vi "CRC_TESTED.vi"() -> ()   [LabVIEW 2019]
panel:
  out "Numeric 7":u16 format="%b"
  out "Numeric":u16 format="%b"
  out "CRC =   5":u16 format="%x"
  out "CRC =   4":u16 format="%b"
  out "CRC =   3":u16 format="%b"
  out "CRC =   2":u16 format="%x"
  in  "DATA PACKET":string
  out "CRC =":u16 format="%x"
  # "1100 0110 1100 1100"
  # "Polynom X16+X12+X5+1"
  # "Felica and 14443 Type A - GOOD"
  # "15693 and 14443 Type B"
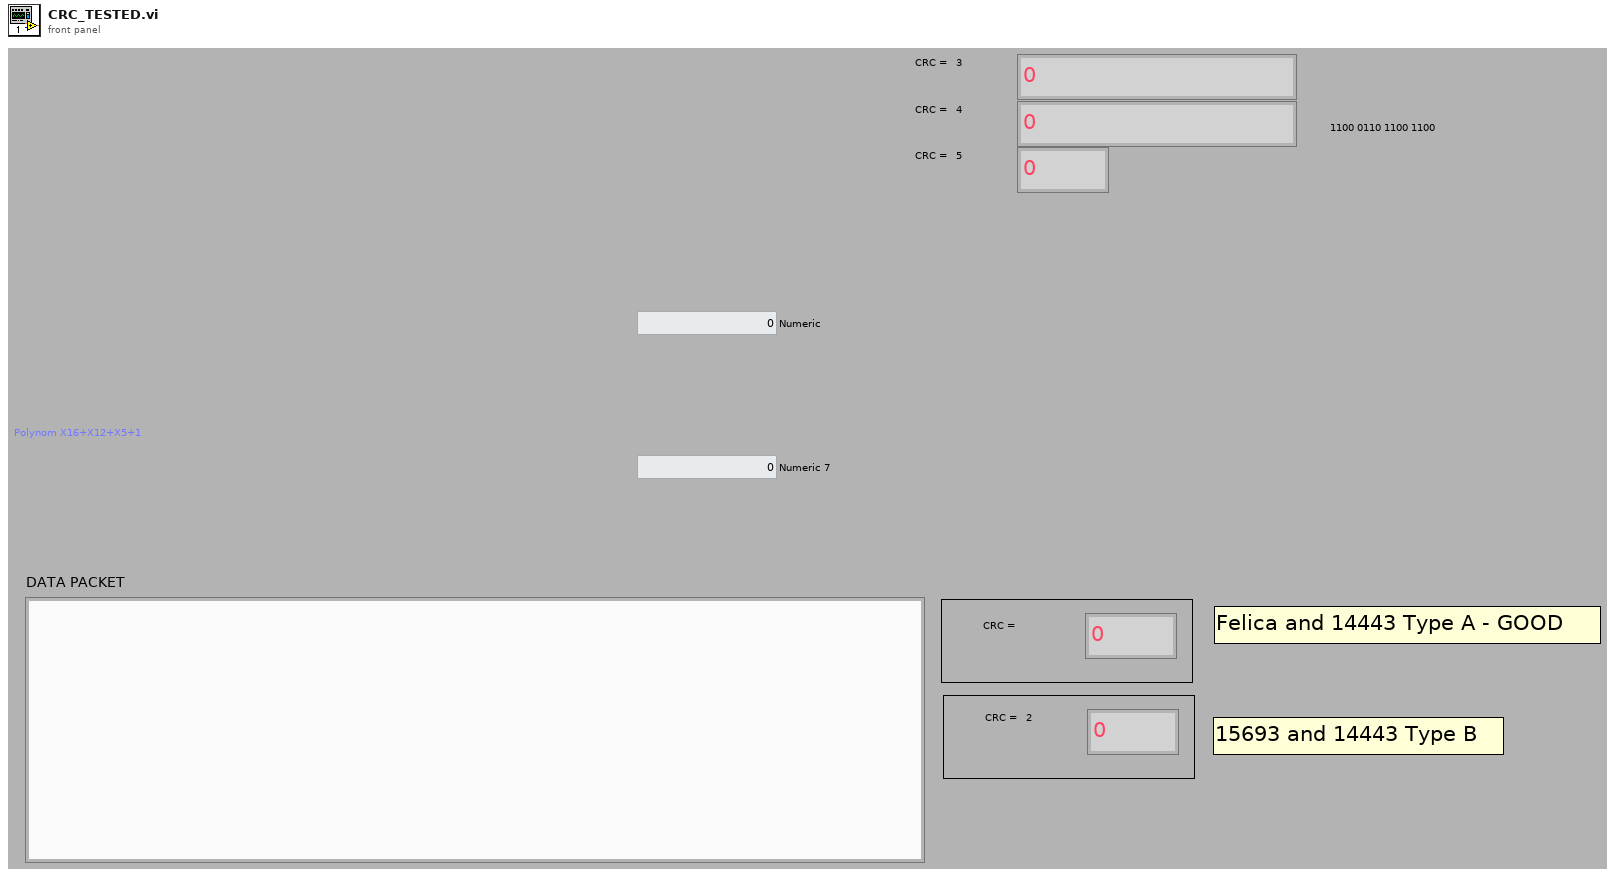
[diagram p1: front panel]
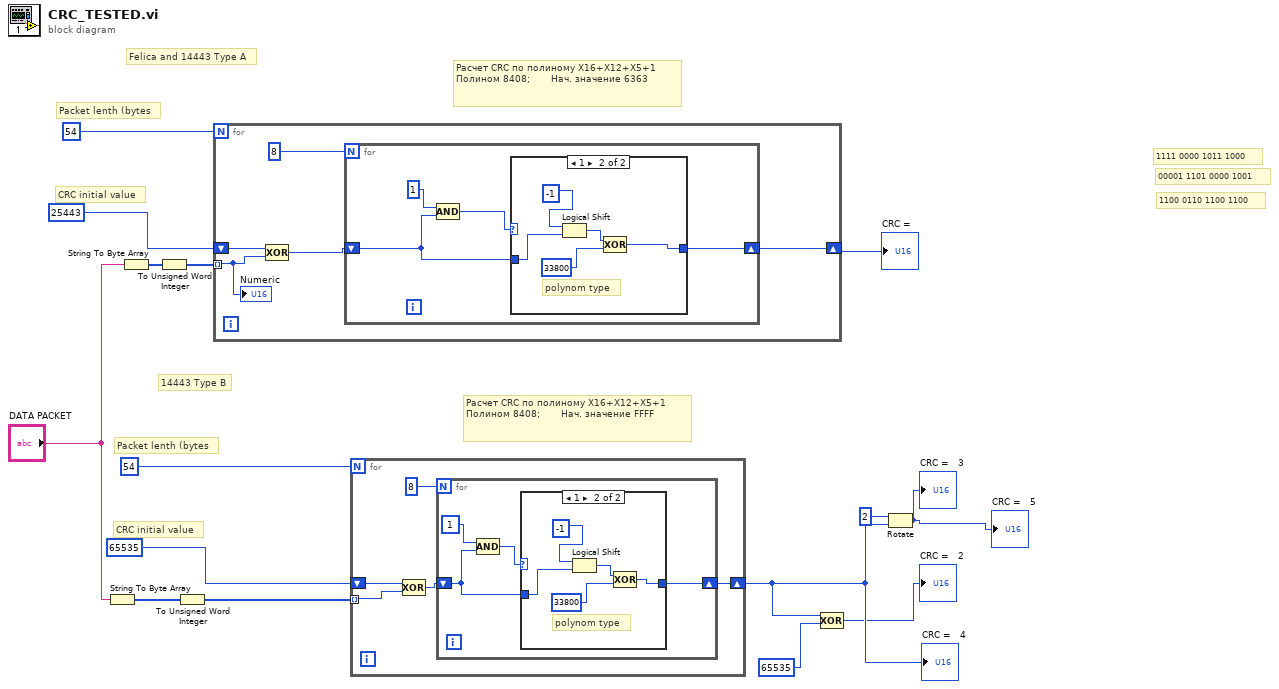
[diagram p0: block diagram]
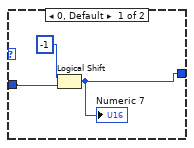
[diagram p2: hidden frame]
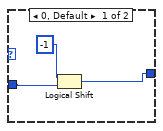
[diagram p3: hidden frame]
diagram:
  # "1111 0000 1011 1000"
  # "1100 0110 1100 1100"
  # "00001 1101 0000 1001"
  # "Felica and 14443 Type A"
  # "Packet lenth (bytes"
  # "CRC initial value"
  # "Расчет CRC по полиному X16+X12+X5+1\nПолином 8408;       Нач. значение 6363"
  # "14443 Type B"
  # "Packet lenth (bytes"
  # "CRC initial value"
  # "Расчет CRC по полиному X16+X12+X5+1\nПолином 8408;       Нач. значение FFFF"
  n1 = String To Byte Array(string="DATA PACKET") -> (unsigned byte array=w5:u8[])
  n2 = String To Byte Array(string="DATA PACKET") -> (unsigned byte array=w10:u8[])
  n3 = To Unsigned Word Integer(number=w10) -> (unsigned 16bit integer=w9:u16[])
  n4 = To Unsigned Word Integer(number=w5) -> (unsigned 16bit integer=w8:u16[])
  n5 = for {
    N: 54 -> [_]
    shift-right: [w16] -> w4
    shift-left: u16 25443 -> [w18]
    tunnel: w9 -> [w19] mode=indexing
    n6 = Compound Arithmetic op=XOR(w18, w19) -> (w17:u32)
    n7 = for {
      N: 8 -> [_]
      shift-right: [w23] -> w16
      shift-left: w17 -> [w22]
      n8 = Compound Arithmetic op=AND(u16 1, w22) -> (w21:u32)
      n9 = case shown="1" w21 {
        tunnel: [w25 w28] -> w23
        tunnel: w22 -> [w26 w31]
        frame 0, Default {
          n10 = Logical Shift(y=i16 -1, x=w26) -> (x << y=w25:u32)
          "Numeric 7" <- w25
        }
        frame 1 {
          # "polynom type"
          n11 = Logical Shift(y=i16 -1, x=w31) -> (x << y=w30:u32)
          n12 = Compound Arithmetic op=XOR(w30, u32 33800) -> (w28:u32)
        }
      }
    }
    "Numeric" <- w19
  }
  "CRC =" <- w4
  n13 = for {
    N: 54 -> [_]
    shift-right: [w34] -> w3
    shift-left: u16 65535 -> [w35]
    tunnel: w8 -> [w33] mode=indexing
    n14 = Compound Arithmetic op=XOR(w35, w33) -> (w36:u32)
    n15 = for {
      N: 8 -> [_]
      shift-right: [w40] -> w34
      shift-left: w36 -> [w39]
      n16 = Compound Arithmetic op=AND(u16 1, w39) -> (w38:u32)
      n17 = case shown="1" w38 {
        tunnel: [w43 w48] -> w40
        tunnel: w39 -> [w42 w45]
        frame 0, Default {
          n18 = Logical Shift(y=i16 -1, x=w42) -> (x << y=w43:u32)
        }
        frame 1 {
          # "polynom type"
          n19 = Logical Shift(y=i16 -1, x=w45) -> (x << y=w47:u32)
          n20 = Compound Arithmetic op=XOR(w47, u32 33800) -> (w48:u32)
        }
      }
    }
  }
  "CRC =   4" <- w3
  n21 = Compound Arithmetic op=XOR(w3, u16 65535) -> (→"CRC =   2":u32)
  n22 = Rotate(1:w3, 2:i16 2 ("y")) -> (0:→"CRC =   3" →"CRC =   5":u32)
